vi "gausian.vi"(1 "Amplitud":dbl, 2 "sigma":sgl, 3 "miu":sgl, 4 "x":sgl) -> (0 "out":dbl)   [LabVIEW 2010]
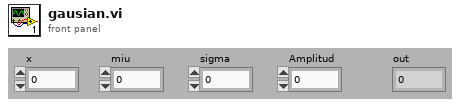
[diagram p1: front panel]
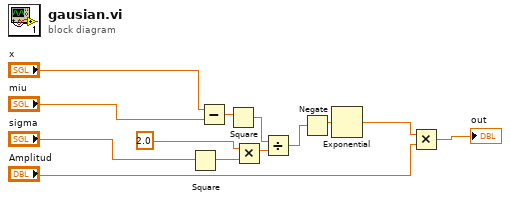
[diagram p0: block diagram]
diagram:
  n1 = Square(x="sigma") -> (x^2=w6:sgl)
  n2 = Subtract(x="x", y="miu") -> (x-y=w3:sgl)
  n3 = Square(x=w3) -> (x^2=w4:sgl)
  n4 = Multiply(x=2.0, y=w6) -> (x*y=w5:dbl)
  n5 = Divide(x=w4, y=w5) -> (x/y=w7:dbl)
  n6 = Negate(x=w7) -> (-x=w2:dbl)
  n7 = Exponential(1:w2) -> (0:w9:dbl)
  n8 = Multiply(x=w9, y="Amplitud") -> (x*y=→"out":dbl)
